vi "DQ subVI.vi"(9 "window (h)":i32, 11 "XY-data":cluster{"X-array":dbl[], "Y-array":dbl[]}) -> (3 "XY-data":cluster{"X-array":dbl[], "Y-array":dbl[]})   [LabVIEW 2019, in "xy_utilities.lvlib"]
doc: "Difference Quotient subVI"
uses:
  xy_utilities.lvlib
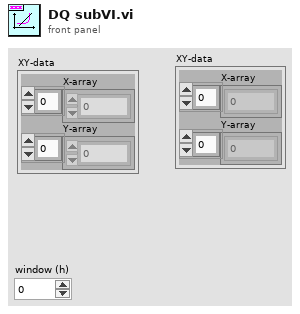
[diagram p1: front panel]
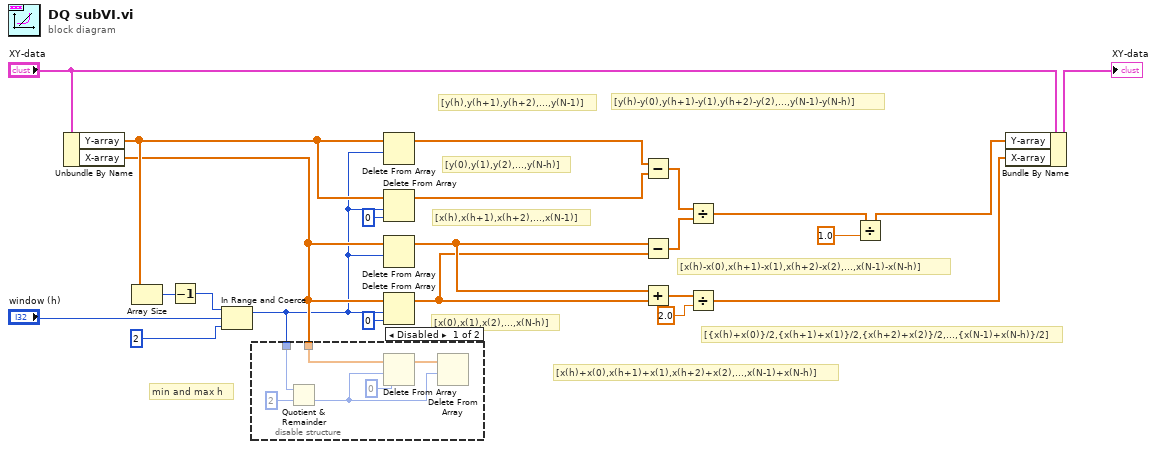
[diagram p0: block diagram]
diagram:
  # "[{x(h)+x(0)}/2,{x(h+1)+x(1)}/2,{x(h+2)+x(2)}/2,...,{x(N-1)+x(N-h)}/2]"
  # "[x(h)+x(0),x(h+1)+x(1),x(h+2)+x(2),...,x(N-1)+x(N-h)]"
  # "[x(0),x(1),x(2),...,x(N-h)]"
  # "[x(h),x(h+1),x(h+2),...,x(N-1)]"
  # "[x(h)-x(0),x(h+1)-x(1),x(h+2)-x(2),...,x(N-1)-x(N-h)]"
  # "[y(h)-y(0),y(h+1)-y(1),y(h+2)-y(2),...,y(N-1)-y(N-h)]"
  # "[y(0),y(1),y(2),...,y(N-h)]"
  # "[y(h),y(h+1),y(h+2),...,y(N-1)]"
  # "min and max h"
  n1 = Unbundle By Name("XY-data") -> ("Y-array"=w12:dbl[], "X-array"=w11:dbl[])
  n2 = Array Size(array=w12) -> (size(s)=w19:i32)
  n3 = Decrement(x=w19) -> (x-1=w20:i32)
  n4 = In Range and Coerce(upper limit=w20, x="window (h)", lower limit=2) -> (coerced(x)=w10:i32)  [unwired: 1 out]
  n5 = disable-structure shown="Disabled" {
    disable-tunnel: w11 -> [w26 _]
    disable-tunnel: w10 -> [w25 _]
    frame Disabled {
      n6 = Quotient & Remainder(x=w25, y=2) -> (floor(x/y)=w24:i32)  [unwired: 1 out]
      n7 = Delete From Array(array=w26, length=w24, index=0) -> (array with subset deleted=w28:dbl[])  [unwired: 1 out]
      n8 = Delete From Array(array=w28, length=w24) -> ()  [unwired: 1 in, 2 out]
    }
    frame Enabled {
    }
  }
  n9 = Delete From Array(array=w12, length=w10) -> (array with subset deleted=w15:dbl[])  [unwired: 1 in, 1 out]
  n10 = Delete From Array(array=w12, length=w10, index=0) -> (array with subset deleted=w16:dbl[])  [unwired: 1 out]
  n11 = Delete From Array(array=w11, length=w10) -> (array with subset deleted=w5:dbl[])  [unwired: 1 in, 1 out]
  n12 = Delete From Array(array=w11, length=w10, index=0) -> (array with subset deleted=w4:dbl[])  [unwired: 1 out]
  n13 = Subtract(x=w15, y=w16) -> (x-y=w13:dbl[])
  n14 = Subtract(x=w5, y=w4) -> (x-y=w9:dbl[])
  n15 = Add(x=w5, y=w4) -> (x+y=w7:dbl[])
  n16 = Divide(x=w13, y=w9) -> (x/y=w2:dbl[])
  n17 = Divide(x=w7, y=2.0) -> (x/y=w6:dbl[])
  n18 = Divide(x=w2, y=1.0) -> (x/y=w1:dbl[])
  n19 = Bundle By Name(cluster="XY-data", "Y-array"=w1, "X-array"=w6) -> (→"XY-data":cluster{"X-array":dbl[], "Y-array":dbl[]})
